vi "Elevator Controller.vi"(2 "error in (no error)":errorcluster, 3 "Command List":T3(array[cluster]), 4 "Boolean Input":u32[](array[numeric])) -> (0 "error out":errorcluster)   [LabVIEW 2018]
uses:
  States.ctl
  Buttons.ctl
  Robot Global Data.vi
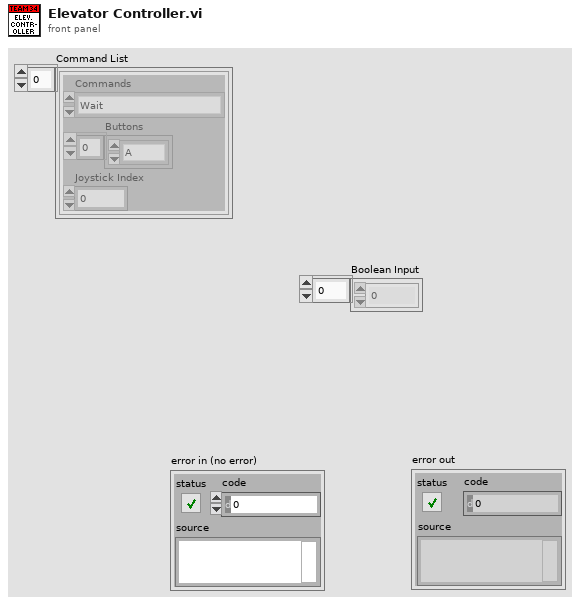
[diagram p1: front panel]
types:
  T1 = typedef "States.ctl" = enum16{"Wait", "Stop", "Limelight Follow", "NavX Reset", "Calibrate Wheels", "Pivot Forward", "Pivot Backward", "Flywheel Forward", "Flywheel Reverse", "FlyDrive Close", "FlyDrive Open", "Pivot Setpoint 0", "Pivot Setpoint 45", "Pivot Setpoint 90", "Low Goal", "Mid Goal", "High Goal", "Low Hatch", "Mid Hatch", "High Hatch", "Vision Track", "Hold Mode", "Pickup", "Dropoff"}
  T2 = typedef "Buttons.ctl" = enum16{"A", "B", "X", "Y", "LB", "RB", "Back", "Start", "LS", "RS"}
  T3 = cluster{"Commands":T1, "Buttons":T2[], "Joystick Index":i32}[]
  T4 = enum16{"Low Hatch", "Low Goal", "Mid Hatch", "Mid Goal", "High Hatch", "High Goal"}
  T5 = enum16{"Open", "Raw Control", "Position Control"}
  T6 = enum16{"Open", "Raw Control", "Position Control", "Autonomous Pickup", "Autonomous Dropoff"}
  T7 = typedef "WPI_EncoderDevRef.ctl" = cluster{"DevStatus":errorcluster, "EncoderIndex":T8, "CounterIndex":T9, "DistancePerCount":dbl, "Decoding Type":T10}
  T8 = typedef "FPGA_EncoderIdx.ctl" = enum8{"Enc 0", "Enc 1", "Enc 2", "Enc 3", "Enc 4", "Enc 5", "Enc 6", "Enc 7", "Invalid"}
  T9 = typedef "FPGA_CounterCtrSystemIndex.ctl" = enum8{"Ctr 0", "Ctr 1", "Ctr 2", "Ctr 3", "Ctr 4", "Ctr 5", "Ctr 6", "Ctr 7", "Invalid"}
  T10 = typedef "WPI_EncoderType.ctl" = enum16{"1x", "2x", "4x"}
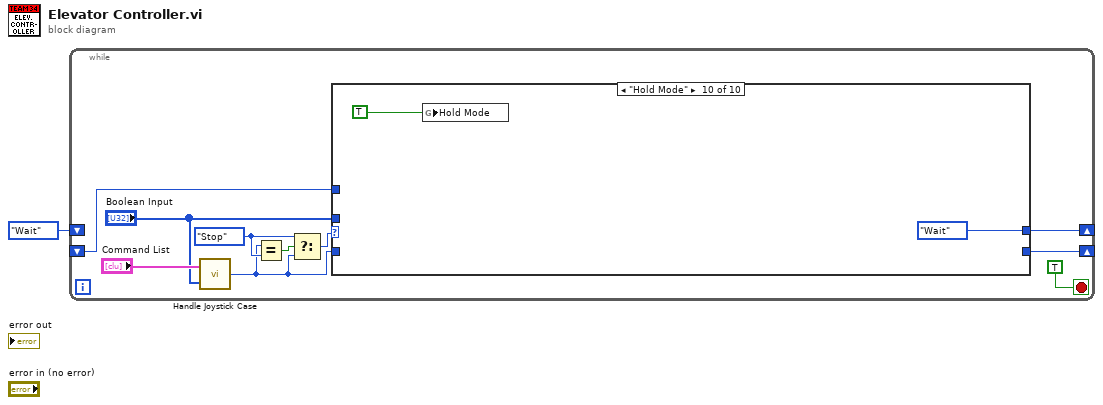
[diagram p0: block diagram]
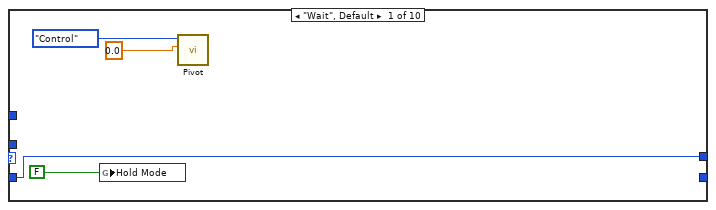
[diagram p2: hidden frame]
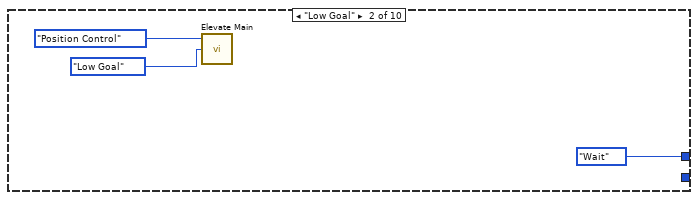
[diagram p3: hidden frame]
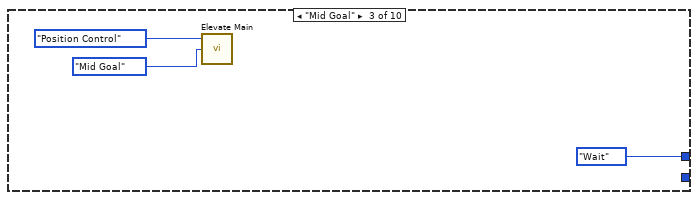
[diagram p4: hidden frame]
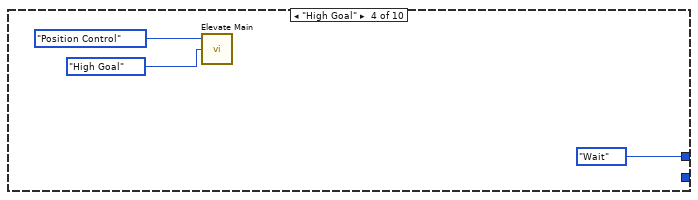
[diagram p5: hidden frame]
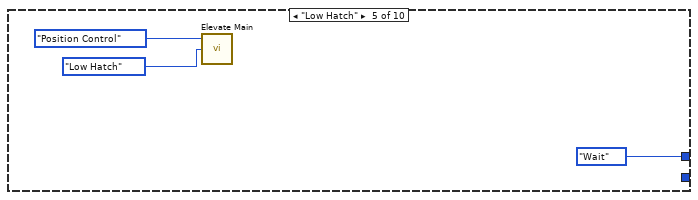
[diagram p6: hidden frame]
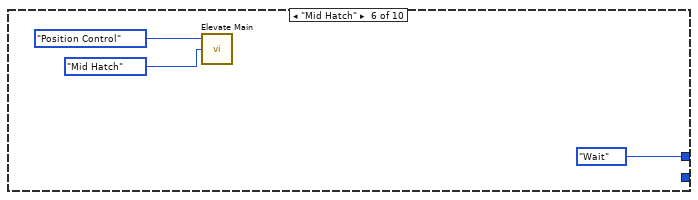
[diagram p7: hidden frame]
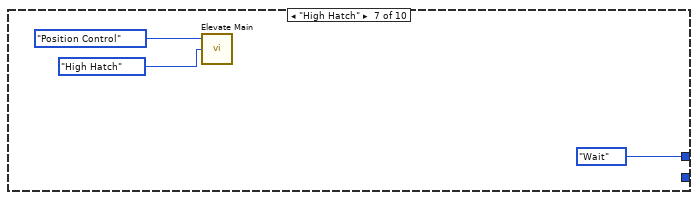
[diagram p8: hidden frame]
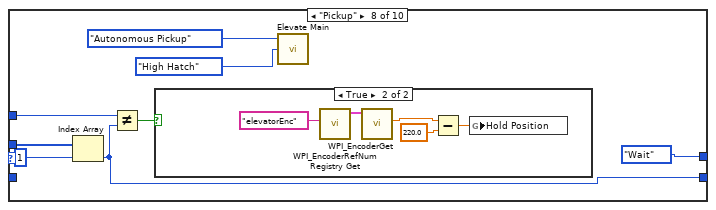
[diagram p9: hidden frame]
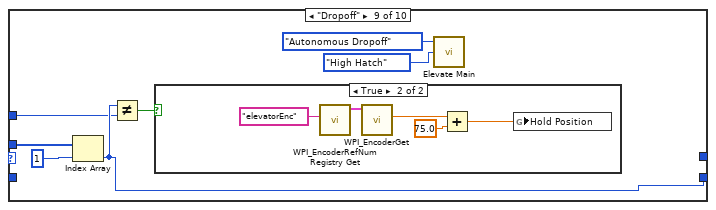
[diagram p11: hidden frame]
diagram:
  n1 = while {
    shift-right: [w7] -> _
    shift-left: States."Wait" ("Commands") -> [_]
    shift-right: [w3] -> _
    shift-left: _ -> [w2]
    stop <- TRUE stop-if-true
    w9 = States."Stop" ("y")
    n2 = call "Handle Joystick Case.vi"("Boolean Input"="Boolean Input", "Command List"="Command List") -> ("Commands"=w6:T1)
    n3 = Equal?(x=w6, y=w9) -> (x = y?=w10:bool)
    n4 = Select(t=w9, s=w10, f=w6) -> (s? t:f=w8:T1)
    n5 = case shown="\"Hold Mode\"" w8 {
      tunnel: [w15 States."Wait" ("Commands") States."Wait" ("Commands") States."Wait" ("Commands") States."Wait" ("Commands") States."Wait" ("Commands") States."Wait" ("Commands") States."Wait" ("Commands") _ States."Wait" ("Commands")] -> w7
      tunnel: w6 -> [w15 _ _ _ _ _ _ _ _ _]
      tunnel: "Boolean Input" -> [_ _ _ _ _ _ _ w38 w52 _]
      tunnel: [_ _ _ _ _ _ _ w37 w51 _] -> w3
      tunnel: w2 -> [_ _ _ _ _ _ _ w36 w50 _]
      frame "Wait", Default {
        n6 = global write "Robot Global Data.vi" "Hold Mode"(FALSE ("Hold Mode")) -> ()
        n7 = call "Pivot.vi"("Output"=0.0, "Enum"=enum16{"SetPoint", "Open", "Control"}."Control") -> ()  [unwired: 10 in]
      }
      frame "Low Goal" {
        n8 = call "Elevate Main.vi"("Level"=T4."Low Goal", "Control Mode"=T5."Position Control") -> ()  [unwired: 2 in]
      }
      frame "Mid Goal" {
        n9 = call "Elevate Main.vi"("Level"=T4."Mid Goal", "Control Mode"=T5."Position Control") -> ()  [unwired: 2 in]
      }
      frame "High Goal" {
        n10 = call "Elevate Main.vi"("Level"=T4."High Goal", "Control Mode"=T5."Position Control") -> ()  [unwired: 2 in]
      }
      frame "Low Hatch" {
        n11 = call "Elevate Main.vi"("Level"=T4."Low Hatch", "Control Mode"=T5."Position Control") -> ()  [unwired: 2 in]
      }
      frame "Mid Hatch" {
        n12 = call "Elevate Main.vi"("Level"=T4."Mid Hatch", "Control Mode"=T5."Position Control") -> ()  [unwired: 2 in]
      }
      frame "High Hatch" {
        n13 = call "Elevate Main.vi"("Level"=T4."High Hatch", "Control Mode"=T5."Position Control") -> ()  [unwired: 2 in]
      }
      frame "Pickup" {
        n14 = Index Array(array=w38, index=1) -> (element=w37:u32)
        n15 = Not Equal?(x=w36, y=w37) -> (x != y?=w35:bool)
        n16 = case shown="True" w35 {
          frame False {
          }
          frame True {
            n17 = call <vilib>:"WPI_EncoderRefNum Registry Get.vi"("refnum name"="elevatorEnc") -> ("EncoderDevRef"=w45:T7)  [unwired: 9 in, 1 out]
            n18 = call <vilib>:"WPI_EncoderGet.vi"("EncoderDevRef"=w45) -> ("Distance"=w44:dbl)  [unwired: 5 in, 5 out]
            n19 = Subtract(x=w44, y=220.0) -> (x-y=w42:dbl)
            n20 = global write "Robot Global Data.vi" "Hold Position"(w42) -> ()
          }
        }
        n21 = call "Elevate Main.vi"("Level"=T4."High Hatch", "Control Mode"=T6."Autonomous Pickup") -> ()  [unwired: 2 in]
      }
      frame "Dropoff" {
        n22 = Index Array(array=w52, index=1) -> (element=w51:u32)
        n23 = Not Equal?(x=w51, y=w50) -> (x != y?=w53:bool)
        n24 = case shown="True" w53 {
          frame False {
          }
          frame True {
            n25 = call <vilib>:"WPI_EncoderRefNum Registry Get.vi"("refnum name"="elevatorEnc") -> ("EncoderDevRef"=w57:T7)  [unwired: 9 in, 1 out]
            n26 = call <vilib>:"WPI_EncoderGet.vi"("EncoderDevRef"=w57) -> ("Distance"=w56:dbl)  [unwired: 5 in, 5 out]
            n27 = Add(x=w56, y=75.0) -> (x+y=w54:dbl)
            n28 = global write "Robot Global Data.vi" "Hold Position"(w54) -> ()
          }
        }
        n29 = call "Elevate Main.vi"("Level"=T4."High Hatch", "Control Mode"=T6."Autonomous Dropoff") -> ()  [unwired: 2 in]
      }
      frame "Hold Mode" {
        n30 = global write "Robot Global Data.vi" "Hold Mode"(TRUE ("Hold Mode")) -> ()
      }
    }
  }
